vi "State Process.vi"(8 "error in (no error)":errorcluster, 11 "View Model":T1) -> (0 "error out":errorcluster, 3 "View Model":T1)   [LabVIEW 2017]
doc: "Perform actions specific to a state"
uses:
  View Model/Controls/View Model.ctl
  Error Handler/Controls/Error Model.ctl
  Error Handler/Controls/Error EventData.ctl
  Error Handler/Controls/Error Type.ctl
  Controls/Elevator Model.ctl
  Controls/Elevator Overhead.ctl
  Controls/Elevator States.ctl
  Controls/Elevator Location.ctl
  Controls/Elevator Command Event.ctl
  Controls/Elevator Commands.ctl
  Configuration/Controls/Configuration Model.ctl
  Configuration/Controls/Configuration Data.ctl
  View Model/Controls/Shared Model.ctl
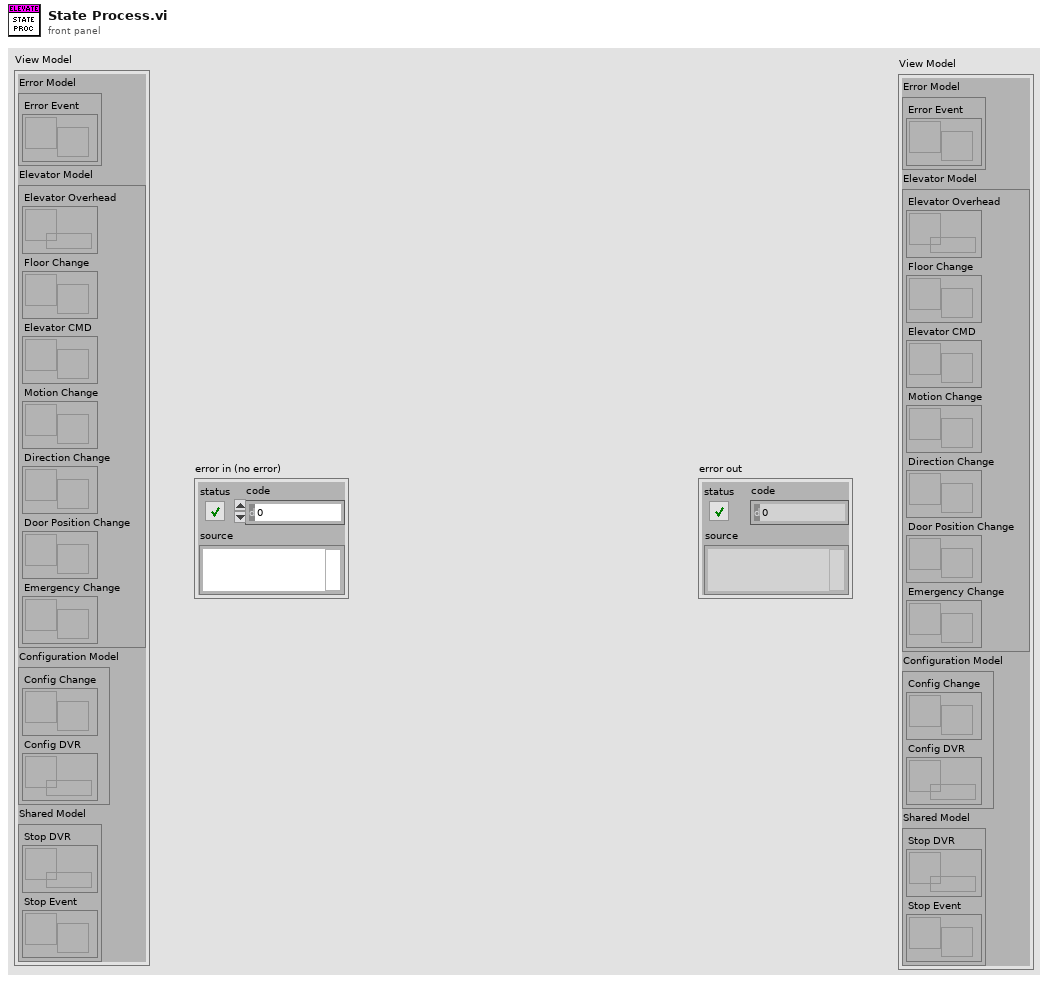
[diagram p1: front panel]
types:
  T1 = typedef "View Model.ctl" = cluster{"Error Model":T2, "Elevator Model":T3, "Configuration Model":T4, "Shared Model":T5}
  T2 = typedef "Error Model.ctl" = cluster{"Error Event":refnum<user-event>}
  T3 = typedef "Elevator Model.ctl" = cluster{"Elevator Overhead":refnum<data-value>, "Floor Change":refnum<user-event>, "Elevator CMD":refnum<user-event>, "Motion Change":refnum<user-event>, "Direction Change":refnum<user-event>, "Door Position Change":refnum<user-event>, "Emergency Change":refnum<user-event>}
  T4 = typedef "Configuration Model.ctl" = cluster{"Config Change":refnum<user-event>, "Config DVR":refnum<data-value>}
  T5 = typedef "Shared Model.ctl" = cluster{"Stop DVR":refnum<data-value>, "Stop Event":refnum<user-event>}
  T6 = typedef "Elevator States.ctl" = enum16{"Idle", "Init", "Open Doors", "Close Doors", "Start Move", "Move", "Finish Move", "Analysis", "Emergency"}
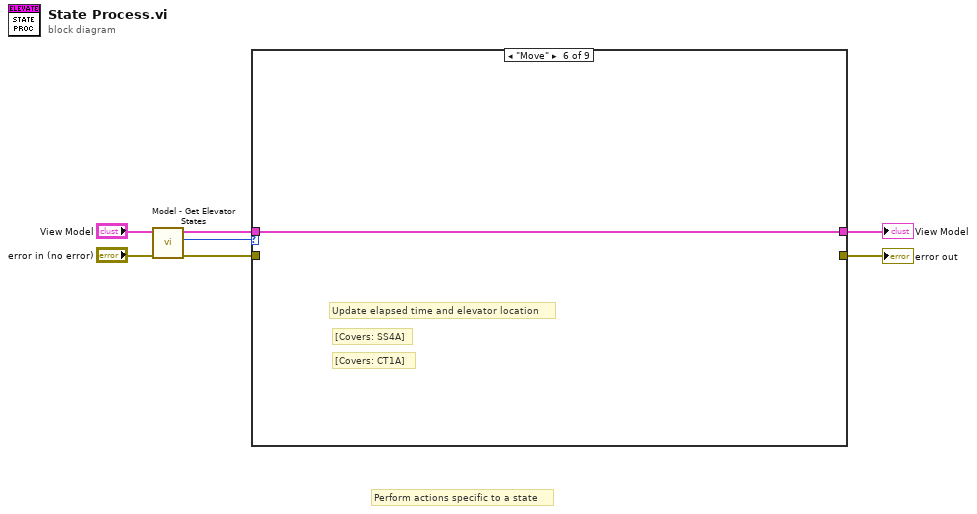
[diagram p0: block diagram]
diagram:
  # "Perform actions specific to a state"
  n1 = call "Model - Get Elevator States.vi"("error in (no error)"="error in (no error)", "View Model"="View Model") -> ("error out"=w4:errorcluster, "Elevator State"=w5:T6, "View Model"=w3:T1)  [unwired: 6 in, 1 out]
  n2 = case shown="\"Move\"" w5 {
    tunnel: w4 -> [w8 _ _ _ _ _ _ _ _]
    tunnel: w3 -> [w9 w10 w11 w12 w13 w14 w15 w16 w17]
    tunnel: [w9 w10 w11 w12 w13 w14 w15 w16 w17] -> w2
    tunnel: [w8 _ _ _ _ _ _ _ _] -> w1
    frame "Idle", Default {
    }
    frame "Init" {
      # "[Covers: NR1]"
      # "Countdown inactivity timer to zero if >0."
      # "[Covers: WS1]"
      # "Maintain initial state defaults"
    }
    frame "Open Doors" {
      # "[Covers: SS1]"
      # "Send digital output to open doors. Fire door open event"
    }
    frame "Close Doors" {
    }
    frame "Start Move" {
    }
    frame "Move" {
      # "[Covers: CT1A]"
      # "[Covers: SS4A]"
      # "Update elapsed time and elevator location"
    }
    frame "Finish Move" {
    }
    frame "Analysis" {
    }
    frame "Emergency" {
    }
  }
  "View Model" <- w2
  "error out" <- w1
